vi "setTerm.vi"(8 "Additional Terminal Options":string, 9 "Height (in)":dbl, 10 "Width (in)":dbl, 11 "String in":string) -> (3 "String out":string, 4 "command":string)   [LabVIEW 2013]
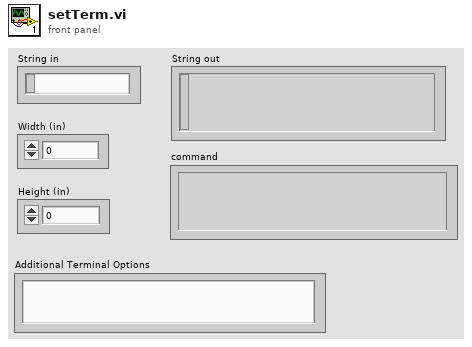
[diagram p1: front panel]
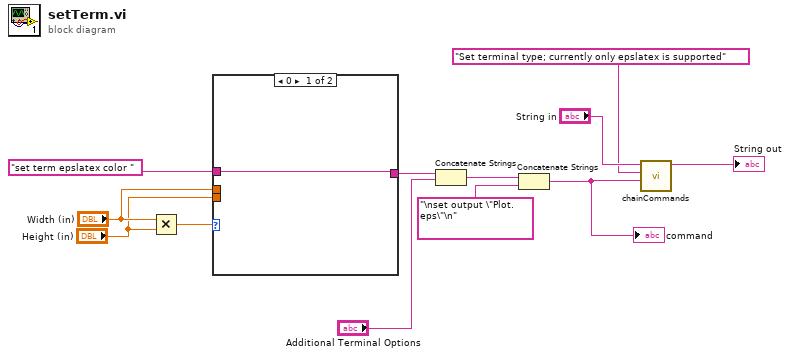
[diagram p0: block diagram]
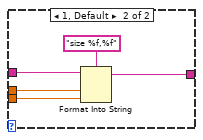
[diagram p2: hidden frame]
diagram:
  n1 = Multiply(x="Width (in)", y="Height (in)") -> (x*y=w8:dbl)
  n2 = case shown="0" w8 {
    tunnel: "set term epslatex color " -> [w13 w17]
    tunnel: [w13 w16] -> w11
    tunnel: "Width (in)" -> [_ w15]
    tunnel: "Height (in)" -> [_ w14]
    frame 0 {
    }
    frame 1, Default {
      n3 = Format Into String(format string="size %f,%f", initial string=w17, w15, w14) -> (resulting string=w16:string)  [unwired: 1 in, 1 out]
    }
  }
  n4 = Concatenate Strings(w11, "Additional Terminal Options") -> (w3:string)
  n5 = Concatenate Strings(w3, "\nset output \"Plot.eps\"\n") -> (w6:string)
  "command" <- w6
  n6 = call "chainCommands.vi"("Command"=w6, "Comments"="Set terminal type; currently only epslatex is supported", "StringIn"="String in") -> ("StringOut"=→"String out":string)  [unwired: 8 in]
